vi "HFRR ADV v06.vi"() -> ()   [LabVIEW 2025] (continued)
            n3605 = Concatenate Strings(w4777, w4776, w4778) -> (w4775:string)
            n3606 = Concatenate Strings(w4767, w4768, w4766) -> (w4769:string)
            n3607 = Concatenate Strings(w4764, w4763, w4765) -> (w4762:string)
            n3608 = Concatenate Strings(w4761, w4773, w4790, w4731) -> (w4737:string)
            n3609 = Concatenate Strings(w4761, w4772, w4783, w4731) -> (w4736:string)
            n3610 = Concatenate Strings(w4761, w4771, w4782, w4731) -> (w4735:string)
            n3611 = Concatenate Strings(w4761, w4770, w4775, w4731) -> (w4734:string)
            n3612 = Concatenate Strings(w4761, w4760, w4769, w4731) -> (w4733:string)
            n3613 = Concatenate Strings(w4761, w4759, w4762, "\"}" ("string")) -> (w4732:string)
            n3614 = Concatenate Strings(w4738, w4737, w4736, w4735, w4734, w4733, w4732, "]}" ("string")) -> (w4729:string)
            n3615 = local read "SEN.RUN HRS"() -> (w4696:dbl)
            n3616 = disable-structure shown="Disabled" {
              frame Disabled {
                n3617 = local read "state"() -> (w4815:string[])
                n3618 = Delete From Array(array=w4815, index=0) -> (array with subset deleted=w4813:string[])  [unwired: 1 in, 1 out]
                n3619 = for {
                  N: 6 -> [_]
                  tunnel: w4813 -> [w4826] mode=indexing
                  tunnel: [w4825] -> w4812 mode=indexing
                  n3620 = Equal?(x=w4826, y="Warning") -> (x = y?=w4822:bool)
                  n3621 = Equal?(x=w4826, y="Healthy") -> (x = y?=w4819:bool)
                  n3622 = Select(t="2" ("y"), s=w4822, f="3" ("y")) -> (s? t:f=w4817:string)
                  n3623 = Select(t="1" ("y"), s=w4819, f=w4817) -> (s? t:f=w4825:string)
                }
                "state1" <- w4812
              }
              frame Enabled {
              }
            }
            n3624 = stacked-sequence {
              tunnel: w4729 -> [w4837 _ _]
              tunnel: [_ _ w4853] -> _
              frame #0 {
                (unwired) FALSE ("convert eol (F)")
                w4839 = enum16{"start", "end", "current"}."start" ("pos mode (0:2)")
                n3625 = local read "Path"() -> (w4833:path)
                n3626 = Path To String(path=w4833) -> (string=w4845:string)
                n3627 = Concatenate Strings(w4845, "\\", "Sensor File Name") -> (w4846:string)
                n3628 = local write "standard output 2"(" ") -> ()
                n3629 = String To Path(string=w4846) -> (path=w4836:path)
                n3630 = call <vilib>:"Open_Create_Replace File.vi"("advisory dialog? (display:T)"=FALSE, "function (open:0)"=T23."create or replace", "file path"=w4836) -> ("error out"=w4849:errorcluster, "refnum"=w4848:refnum<file>)  [unwired: 5 in, 2 out]
                n3631 = Set File Position(refnum=w4848, from (0:start)=w4839, error in=w4849) -> (refnum out=w4829:refnum<file>, error out=w4828:errorcluster)  [unwired: 1 in]
                n3632 = Write to Binary File(file (use dialog)=w4829, data=" ", error in=w4828, 5:FALSE ("prepend array or string size? (T)")) -> (refnum out=w4840:refnum<file>, error out=w4841:errorcluster)  [unwired: 2 in, 1 out]
                n3633 = Set File Position(offset (in bytes) (0)=w4839, refnum=w4840, error in=w4841) -> (refnum out=w4832:refnum<file>, error out=w4831:errorcluster)  [unwired: 1 in]
                n3634 = Write to Binary File(file (use dialog)=w4832, data=w4837, error in=w4831, 5:FALSE ("prepend array or string size? (T)")) -> (error out=w4835:errorcluster)  [unwired: 2 in, 2 out]
                n3635 = flat-sequence {
                  tunnel: w4836 -> [w4851]
                  tunnel: w4835 -> [_]
                  frame #0 {
                    n3636 = call <vilib>:"Read Characters From File.vi"("file path (dialog if empty)"=w4851) -> ("character string"=→"Sensor Health JSON string":string)  [unwired: 5 in, 3 out]
                  }
                }
                "SinglePoint  2" <- w4837
              }
              frame #1 {
              }
              frame #2 {
                (unwired) "\"Stored\": true" ("string")
                n3637 = call <vilib>:"System Exec.vi"("run minimized? (F)"=TRUE, "wait until completion? (T)"=TRUE, "working directory"=path "C:/LAB-IQ-NXT", "command line"="C:\\LAB-IQ-NXT\\JPostH.bat") -> ("standard error"=→"Respose From Server 2":string, "standard output"=w4856:string)  [unwired: 4 in, 2 out]
                "standard output 2" <- w4856
                n3638 = Match Pattern(string=w4856, regular expression="JSONH Check String") -> (match substring=w4854:string, offset past match=w4853:i32)  [unwired: 1 in, 2 out]
                n3639 = Equal?(x=w4854, y="JSONH Check String") -> (x = y?=→"Upload \nConfirmed 2":bool)
              }
            }
            n3640 = Divide(x=w4696, y=3600.0 ("f")) -> (x/y=w4689:dbl)
            n3641 = local read "run time"() -> (w4746:string[])
            n3642 = Round To Nearest(number=w4689) -> (nearest integer value=w4688:dbl)
            n3643 = Number To Decimal String(number=w4688) -> (decimal integer string=w4687:string)  [unwired: 1 in]
            n3644 = Index Array(array="Sensor Information", index (col) #1=0 ("disabled index (col)"), index (col) #2=1 ("index (col)"), index (col) #3=2 ("index (col)"), index (col) #4=3 ("index (col)")) -> (element #1=→"Sensor name":string[], element #2=→"model num":string[], element #3=→"run time":string[], element #4=→"state":string[])  [unwired: 4 in]
            n3645 = Insert Into Array(array=w4746, index=1, new element #1=w4687, new element #2=w4687, new element #3=w4687, new element #4=w4687, new element #5=w4687, new element #6=w4687) -> (w4711:string[])
            "run" <- w4711
            n3646 = local read "out"() -> (w4693:string[])
            n3647 = local read "Sensor Information"() -> (w4713:string[][])
            n3648 = Replace Array Subset(array=w4713, new element #1=w4711, index (col) #1=2 ("disabled index (col)"), new element #2=w4693, index (col) #2=3 ("index (col)")) -> (w4712:string[][])  [unwired: 2 in]
            n3649 = local write "Sensor Information"(w4712) -> ()
          }
        }
        n3650 = case shown="True" w4660 {
          frame False {
          }
          frame True {
            n3651 = Equal?(x="FLAG", y=0.0) -> (x = y?=w4677:bool)
            n3652 = case shown="False" w4677 {
              frame False {
                n3653 = Get Date/Time In Seconds() -> (seconds since 1Jan1904=w4683:timestamp)
                n3654 = local read "START 2"() -> (w4681:dbl)
                n3655 = To Double Precision Float(number=w4683) -> (double precision float=w4682:dbl)
                n3656 = Subtract(x=w4682, y=w4681) -> (x-y=→"SENSOR TIME  2":dbl)
              }
              frame True {
                n3657 = Get Date/Time In Seconds() -> (seconds since 1Jan1904=w4685:timestamp)
                n3658 = To Double Precision Float(number=w4685) -> (double precision float=→"START 2":dbl)
                n3659 = local write "FLAG"(100.0 ("FLAG")) -> ()
              }
            }
          }
        }
        n3660 = disable-structure shown="Disabled" {
          disable-tunnel: w4663 -> [w4672 _]
          disable-tunnel: [w4671 _] -> w4662
          frame Disabled {
            n3661 = local read "Json St Flg"() -> (w4670:bool)
            n3662 = case shown="True" w4670 {
              tunnel: w4672 -> [w4673 w4675]
              tunnel: [w4673 w4674] -> w4671
              frame False {
              }
              frame True {
                n3663 = Increment(x=w4675) -> (x+1=w4674:dbl)
                "T cycle" <- w4674
                n3664 = local write "Json St Flg"(FALSE ("Json St Flg")) -> ()
              }
            }
          }
          frame Enabled {
          }
        }
        n3665 = local read "Quit"() -> (w4657:bool)
      }
    }
    frame Enabled {
    }
  }
  n3666 = stacked-sequence {
    tunnel: [w5055] -> w26
    frame #0 {
      w5055 = FALSE ("Upload \nConfirmed")
      n3667 = local write "Upload \nConfirmed"(w5055) -> ()
      n3668 = local write "St Str"("") -> ()
    }
  }
  n3669 = disable-structure shown="Disabled" {
    disable-tunnel: w26 -> [w5056 _]
    frame Disabled {
      n3670 = case shown="True" {
        selector: _ -> [_ _]
        tunnel: w5056 -> [_ w5057]
        frame False {
        }
        frame True {
          n3671 = while {
            tunnel: [w5063] -> _
            tunnel: w5057 -> [_]
            i -> [w5063]
            stop <- w5058 stop-if-true
            n3672 = local read "Json End Flg"() -> (w5062:bool)
            n3673 = Wait (ms)(milliseconds to wait=u32 20 ("Refresh Rate (ms)")) -> ()  [unwired: 1 out]
            n3674 = local read "refresh flag"() -> (w5059:bool)
            n3675 = local read "RUN"() -> (w5060:bool)
            n3676 = And(x=w5060, y=w5059) -> (x .and. y?=w5061:bool)
            n3677 = Or(x=w5061, y=w5062) -> (x .or. y?=w5064:bool)
            "AR Led" <- w5064
            n3678 = case shown="True" w5064 {
              frame False {
              }
              frame True {
                w5081 = "\",\""
                n3679 = local read "UUID"() -> (w5079:string)
                n3680 = local write "refresh flag"(FALSE ("refresh flag")) -> ()
                n3681 = local read "time"() -> (w5068:dbl)
                n3682 = Multiply(x=w5068, y=60.0) -> (x*y=w5067:dbl)
                n3683 = Concatenate Strings("UUID\" : \"", w5079, "\"}") -> (w5082:string)
                n3684 = Number To Fractional String(number=w5067, width (-)=i16 10, precision (6)=i16 4) -> (F-format string=w5096:string)  [unwired: 1 in]
                n3685 = Concatenate Strings("{", "\"Time\":\"", w5096, w5081) -> (w5091:string)
                n3686 = stacked-sequence {
                  tunnel: w5081 -> [w5144 w5152 w5159 w5167 w5175 w5184 w5191]
                  tunnel: [w5145 _ _ _ _ _ _] -> w5095
                  tunnel: [_ w5153 _ _ _ _ _] -> w5094
                  tunnel: [_ _ w5160 _ _ _ _] -> w5093
                  tunnel: [_ _ _ w5169 _ _ _] -> w5092
                  tunnel: w5082 -> [_ _ _ _ _ _ w5202]
                  tunnel: [_ _ _ _ _ _ w5201] -> w5078
                  tunnel: [_ _ _ _ _ w5181 _] -> w5077
                  tunnel: [_ _ _ _ w5174 _ _] -> w5076
                  frame #0 {
                    n3687 = local read "NORMAL LOAD"() -> (w5143:dbl)
                    n3688 = Number To Fractional String(number=w5143, width (-)=i16 10, precision (6)=i16 4) -> (F-format string=w5146:string)  [unwired: 1 in]
                    n3689 = Concatenate Strings("NormalLoad\":\"", w5146, w5144) -> (w5145:string)
                  }
                  frame #1 {
                    n3690 = local read "Temp"() -> (w5151:dbl)
                    n3691 = Number To Fractional String(number=w5151, width (-)=i16 10, precision (6)=i16 4) -> (F-format string=w5154:string)  [unwired: 1 in]
                    n3692 = Concatenate Strings("Temperature\":\"", w5154, w5152) -> (w5153:string)
                  }
                  frame #2 {
                    n3693 = local read "cof"() -> (w5157:dbl)
                    n3694 = Number To Fractional String(number=w5157, width (-)=i16 10, precision (6)=i16 4) -> (F-format string=w5161:string)  [unwired: 1 in]
                    n3695 = Concatenate Strings("FrictionalForce\":\"", w5161, w5159) -> (w5160:string)
                  }
                  frame #3 {
                    n3696 = local read "Set Hz"() -> (w5165:dbl)
                    n3697 = Multiply(x=w5165, y=60.0) -> (x*y=w5164:dbl)
                    n3698 = Number To Fractional String(number=w5164, width (-)=i16 10, precision (6)=i16 4) -> (F-format string=w5170:string)  [unwired: 1 in]
                    n3699 = Concatenate Strings("Speed\":\"", w5170, w5167) -> (w5169:string)
                  }
                  frame #4 {
                    n3700 = local read "Stroke Ln"() -> (w5173:dbl)
                    n3701 = Number To Fractional String(number=w5173, width (-)=i16 10, precision (6)=i16 4) -> (F-format string=w5177:string)  [unwired: 1 in]
                    n3702 = Concatenate Strings("LinearDeformation\":\"", w5177, w5175) -> (w5174:string)
                  }
                  frame #5 {
                    n3703 = local read "AIR TEMP"() -> (w5180:dbl)
                    n3704 = local read "Json St Flg"() -> (w5182:bool)
                    n3705 = local read "Json End Flg"() -> (w5183:bool)
                    n3706 = Number To Fractional String(number=w5180, width (-)=i16 10, precision (6)=i16 4) -> (F-format string=w5186:string)  [unwired: 1 in]
                    n3707 = Concatenate Strings("Vibration\":\"", w5186, w5184) -> (w5181:string)
                    n3708 = And(x=w5182, y=w5183) -> ()  [unwired: 1 out]
                  }
                  frame #6 {
                    n3709 = local read "Json End Flg"() -> (w5190:bool)
                    n3710 = Get Date/Time In Seconds() -> (seconds since 1Jan1904=w5198:timestamp)
                    n3711 = local read "Json St Flg"() -> (w5189:bool)
                    n3712 = To Double Precision Float(number=w5198) -> (double precision float=w5197:dbl)
                    n3713 = Subtract(x=w5197, y=2082844800.0) -> (x-y=w5195:dbl)
                    n3714 = Number To Fractional String(number=w5195, width (-)=i16 12, precision (6)=i16 0) -> (F-format string=w5192:string)  [unwired: 1 in]
                    n3715 = case shown="True" w5190 {
                      tunnel: ["" w5205] -> w5199
                      tunnel: w5192 -> [_ w5206]
                      tunnel: w5191 -> [_ w5204]
                      frame False {
                      }
                      frame True {
                        n3716 = local write "Json End Flg"(FALSE ("Json St Flg")) -> ()
                        n3717 = Concatenate Strings("End\": \"", w5206, w5204) -> (w5205:string)
                      }
                    }
                    n3718 = case shown="True" w5189 {
                      tunnel: [w5209 w5212] -> w5200
                      tunnel: w5192 -> [_ w5213]
                      tunnel: w5191 -> [_ w5210]
                      frame False {
                        n3719 = local read "St Str"() -> (w5209:string)
                      }
                      frame True {
                        n3720 = Concatenate Strings("Start\":\"", w5213, w5210) -> (w5212:string)
                        "St Str" <- w5212
                        n3721 = local write "Json St Flg"(FALSE ("Json St Flg")) -> ()
                      }
                    }
                    n3722 = Concatenate Strings(w5200, w5199, w5202) -> (w5201:string)
                  }
                }
                n3723 = local read "FILE"() -> (w5070:string)
                n3724 = Concatenate Strings("\",\"OperatorID\":\"" ("string"), "Operator ID") -> (w5073:string)
                n3725 = Concatenate Strings("\",\"DatasetTitle\":\"" ("string"), w5070) -> (w5072:string)
                n3726 = Concatenate Strings("\",\"SerialNumber\":\"" ("string"), "Serial No") -> (w5102:string)
                n3727 = Concatenate Strings("\",\"ModelNumber\":\"" ("string"), "Model No") -> (w5101:string)
                n3728 = Concatenate Strings(w5102, w5101) -> (w5084:string)
                n3729 = Concatenate Strings("{\"SecretKey\":\"", "Secret Key", w5084, w5073, w5072, "\",\"Samples\":[") -> (w5089:string)
                n3730 = Concatenate Strings(w5091, w5095, w5094, w5093, w5092, w5076, w5077, w5078) -> (w5090:string)
                n3731 = Concatenate Strings(w5089, w5090, "]}") -> (w5088:string)
                n3732 = stacked-sequence {
                  tunnel: w5088 -> [w5117 _ _]
                  tunnel: [_ _ w5134] -> _
                  frame #0 {
                    (unwired) FALSE ("convert eol (F)")
                    w5119 = enum16{"start", "end", "current"}."start" ("pos mode (0:2)")
                    n3733 = Path To String(path="Path") -> (string=w5125:string)
                    n3734 = Concatenate Strings(w5125, "\\", "Data File Name") -> (w5127:string)
                    n3735 = local write "standard output"(" ") -> ()
                    n3736 = String To Path(string=w5127) -> (path=w5116:path)
                    n3737 = call <vilib>:"Open_Create_Replace File.vi"("advisory dialog? (display:T)"=FALSE, "function (open:0)"=T23."create or replace", "file path"=w5116) -> ("error out"=w5130:errorcluster, "refnum"=w5129:refnum<file>)  [unwired: 5 in, 2 out]
                    n3738 = Set File Position(refnum=w5129, from (0:start)=w5119, error in=w5130) -> (refnum out=w5110:refnum<file>, error out=w5109:errorcluster)  [unwired: 1 in]
                    n3739 = Write to Binary File(file (use dialog)=w5110, data=" ", error in=w5109, 5:FALSE ("prepend array or string size? (T)")) -> (refnum out=w5120:refnum<file>, error out=w5121:errorcluster)  [unwired: 2 in, 1 out]
                    n3740 = Set File Position(offset (in bytes) (0)=w5119, refnum=w5120, error in=w5121) -> (refnum out=w5113:refnum<file>, error out=w5112:errorcluster)  [unwired: 1 in]
                    n3741 = Write to Binary File(file (use dialog)=w5113, data=w5117, error in=w5112, 5:FALSE ("prepend array or string size? (T)")) -> (error out=w5115:errorcluster)  [unwired: 2 in, 2 out]
                    n3742 = flat-sequence {
                      tunnel: w5116 -> [w5132]
                      tunnel: w5115 -> [_]
                      frame #0 {
                        n3743 = call <vilib>:"Read Characters From File.vi"("file path (dialog if empty)"=w5132) -> ("character string"=→"JSON string":string)  [unwired: 5 in, 3 out]
                      }
                    }
                    "SinglePoint" <- w5117
                  }
                  frame #1 {
                  }
                  frame #2 {
                    (unwired) "\"Stored\": true" ("string")
                    n3744 = call <vilib>:"System Exec.vi"("run minimized? (F)"=TRUE, "wait until completion? (T)"=TRUE, "working directory"=path "C:/LAB-IQ-NXT", "command line"="C:\\LAB-IQ-NXT\\JPost.bat") -> ("standard error"=→"Respose From Server":string, "standard output"=w5137:string)  [unwired: 4 in, 2 out]
                    "standard output" <- w5137
                    n3745 = Match Pattern(string=w5137, regular expression="JSON Check String") -> (match substring=w5135:string, offset past match=w5134:i32)  [unwired: 1 in, 2 out]
                    n3746 = Equal?(x=w5135, y="JSON Check String") -> (x = y?=→"Upload \nConfirmed":bool)
                  }
                }
              }
            }
            n3747 = local read "Quit"() -> (w5058:bool)
          }
        }
      }
    }
    frame Enabled {
    }
  }
  n3748 = disable-structure shown="Disabled" {
    disable-tunnel: _ -> [w5220 _]
    frame Disabled {
      n3749 = while {
        shift-right: [w5228] -> w5216
        shift-left: _ -> [w5229]
        shift-right: [w5226] -> w5217
        shift-left: errorcluster {"status"=TRUE, "code"=0, "source"="Init"} ("error out") -> [w5227]
        shift-right: [w5224] -> _
        shift-left: "" -> [w5225]
        tunnel: [w5222] -> _
        tunnel: w5220 -> [_]
        i -> [w5222]
        stop <- w5221 stop-if-true
        n3750 = flat-sequence {
          tunnel: [w5230] -> w5223
          frame #0 {
            n3751 = Wait (ms)(milliseconds to wait=10.0 ("Delay")) -> (millisecond timer value=w5230:u32)
          }
        }
        n3752 = case shown="No Error" w5227 {
          selector: w5227 -> [w5263 w5385]
          tunnel: [w5245 w5387] -> w5228
          tunnel: [w5244 w5386] -> w5226
          tunnel: w5229 -> [w5264 w5379]
          tunnel: w5225 -> [w5243 w5378]
          tunnel: [w5242 w5378] -> w5224
          tunnel: w5223 -> [_ _]
          frame No Error {
            n3753 = Concatenate Strings("COMMAND", "\r", "\n") -> (w5254:string)
            n3754 = case shown="True" "Measure" {
              tunnel: w5264 -> [w5290 w5297]
              tunnel: w5263 -> [w5289 w5296]
              tunnel: [w5290 w5295] -> w5262
              tunnel: [w5289 w5294] -> w5241
              tunnel: w5254 -> [_ w5293]
              frame False {
              }
              frame True {
                n3755 = VISA Write(VISA resource name=w5297, write buffer=w5293, error in (no error)=w5296) -> (VISA resource name out=w5295:refnum<visa-resource-name>, error out=w5294:errorcluster)  [unwired: 1 out]
                n3756 = local write "Read String"("") -> ()
                n3757 = local write "Measure"(FALSE) -> ()
              }
            }
            n3758 = property class="Instr"(reference=w5262, error in=w5241) -> (reference out=w5261:refnum<visa-resource-name>, error out=w5260:errorcluster, "Serial Settings:Number of Bytes at Serial Port"=w5259:u32)
            n3759 = Greater?(x=w5259, y=u32 100) -> (0:w5257:bool)
            n3760 = case shown="True" w5257 {
              tunnel: w5261 -> [w5300 w5325]
              tunnel: w5260 -> [w5299 w5324]
              tunnel: w5259 -> [_ w5323]
              tunnel: [w5300 w5322] -> w5247
              tunnel: [w5299 w5321] -> w5246
              tunnel: w5243 -> [w5298 w5320]
              tunnel: [w5298 ""] -> w5242
              frame False {
              }
              frame True {
                w5310 = u32 6 ("y")
                # "Page 84 of \nmanual"
                n3761 = VISA Read(VISA resource name=w5325, byte count=w5323, error in (no error)=w5324) -> (VISA resource name out=w5322:refnum<visa-resource-name>, read buffer=w5318:string, error out=w5321:errorcluster)  [unwired: 1 out]
                n3762 = while {
                  tunnel: w5318 -> [w5374]
                  tunnel: [w5370] -> w5312 mode=indexing
                  tunnel: [w5364] -> w5316 mode=indexing
                  tunnel: [w5362] -> _
                  i -> [w5362]
                  stop <- w5367 stop-if-true
                  n3763 = String Subset(string=w5374, offset (0)=w5362) -> (substring=w5369:string)  [unwired: 1 in]
                  n3764 = String To Byte Array(string=w5369) -> (unsigned byte array=w5373:u8[])
                  n3765 = String Length(string=w5369) -> (length=w5368:i32)
                  n3766 = Index Array(array=w5373) -> (element=w5372:u8)  [unwired: 1 in]
                  n3767 = Equal To 0?(x=w5368) -> (x = 0?=w5367:bool)
                  n3768 = Number To Boolean Array(number=w5372) -> (Boolean array=w5366:bool[])
                  n3769 = Reverse 1D Array(array=w5366) -> (reversed array=w5365:bool[])
                  n3770 = And(x=w5366, y=bool[] [FALSE, FALSE, FALSE, FALSE, FALSE, FALSE, TRUE, TRUE] ("Boolean array")) -> (x .and. y?=w5370:bool[])
                  n3771 = And(x=w5365, y=bool[] [FALSE, FALSE, TRUE, TRUE, TRUE, TRUE, TRUE, TRUE] ("Boolean array")) -> (x .and. y?=w5364:bool[])
                }
                n3772 = Concatenate Strings(w5320, w5318) -> (→"Read String":string)
                n3773 = while {
                  tunnel: w5312 -> [w5361] mode=indexing
                  tunnel: [w5357] -> w5315
                  i -> [w5357]
                  stop <- w5358 stop-if-true
                  n3774 = Search 1D Array(1D array=w5361, element=TRUE) -> (index of element=w5359:i32)  [unwired: 1 in]
                  n3775 = Less Than 0?(x=w5359) -> (x < 0?=w5358:bool)
                }
                n3776 = Delete From Array(array=w5316, length=w5315, index (row)=0) -> (array with subset deleted=w5311:bool[][])  [unwired: 1 in, 1 out]
                n3777 = Array Size(array=w5311) -> (size(s)=w5313:i32[])
                n3778 = Index Array(array=w5313) -> (element=w5305:i32)  [unwired: 1 in]
                n3779 = Greater?(x=w5305, y=w5310) -> (0:w5308:bool)
                n3780 = Subtract(x=w5305, y=w5310) -> (x-y=w5309:u32)
                n3781 = Select(t=w5309, s=w5308, f=u32 0) -> (s? t:f=w5306:u32)
                n3782 = while {
                  tunnel: w5311 -> [w5344]
                  tunnel: [w5346] -> w5304 mode=indexing
                  tunnel: w5306 -> [w5328]
                  i -> [w5345]
                  stop <- w5343 stop-if-true
                  w5335 = 6 ("index")
                  w5334 = 2 ("length")
                  # "Page 65 of \nmanual"
                  n3783 = Multiply(x=u32 3 ("y"), y=w5345) -> (x*y=w5342:u32)
                  n3784 = Divide(x=u32 102 ("y"), y=u32 65520) -> (x/y=w5352:dbl)
                  n3785 = Greater Or Equal?(x=w5342, y=w5328) -> (x >= y?=w5343:bool)
                  n3786 = Index Array(array=w5344, index (row) #1=w5342) -> (element #1=w5340:bool[], element #2=w5339:bool[], element #3=w5338:bool[])  [unwired: 5 in]
                  n3787 = Reverse 1D Array(array=w5340) -> (reversed array=w5333:bool[])
                  n3788 = Reverse 1D Array(array=w5339) -> (reversed array=w5337:bool[])
                  n3789 = Reverse 1D Array(array=w5338) -> (reversed array=w5336:bool[])
                  n3790 = Delete From Array(array=w5333, length=w5334, index=w5335) -> (array with subset deleted=w5329:bool[])  [unwired: 1 out]
                  n3791 = Delete From Array(array=w5337, length=w5334, index=w5335) -> (array with subset deleted=w5330:bool[])  [unwired: 1 out]
                  n3792 = Delete From Array(array=w5336, length=w5334, index=w5335) -> (array with subset deleted=w5331:bool[])  [unwired: 1 out]
                  n3793 = Insert Into Array(array=bool[] [] ("Boolean array"), new element #1=w5329, new element #2=w5330, new element #3=w5331) -> (w5332:bool[])  [unwired: 1 in]
                  n3794 = Boolean Array To Number(Boolean array=w5332) -> (number=w5341:u32)
                  n3795 = Multiply(x=w5352, y=w5341) -> (x*y=w5351:dbl)
                  n3796 = Decrement(x=w5351) -> (x-1=w5350:dbl)
                  n3797 = Divide(x=w5350, y=u32 100) -> (x/y=w5348:dbl)
                  n3798 = Multiply(x=w5348, y=u32 10) -> (x*y=w5346:dbl)
                }
                n3799 = Delete From Array(array=w5304) -> (array with subset deleted=w5303:dbl[])  [unwired: 2 in, 1 out]
                "Waveform Graph 5" <- w5303
                "Waveform Chart 3" <- w5303
                n3800 = call-poly <vilib>:"Mean.vi"("X"=w5303) -> ("mean"=w5302:dbl)  [unwired: 1 out]
                "Measure_LDS" <- w5302
                n3801 = case shown="True" "Zero 4" {
                  tunnel: w5302 -> [_ w5327]
                  frame False {
                  }
                  frame True {
                    n3802 = local write "Zero 4"(FALSE ("Zero 4")) -> ()
                    "z_measure" <- w5327
                  }
                }
              }
            }
            n3803 = local read "Measure_LDS"() -> (w5237:dbl)
            n3804 = local read "Disp (mm)"() -> (w5236:dbl)
            n3805 = local read "Boolean 7"() -> (w5235:bool)
            n3806 = local read "Boolean 8"() -> (w5234:bool)
            n3807 = case shown="True" "Boolean 8" {
              tunnel: w5236 -> [_ w5267]
              tunnel: w5237 -> [_ w5266]
              frame False {
              }
              frame True {
                n3808 = local read "Captured Values 2"() -> (w5270:dbl[][])
                n3809 = Build Array(w5267, w5266) -> (w5265:dbl[])
                n3810 = Build Array (concatenate)(w5270, w5265) -> (w5268:dbl[][])
                n3811 = local write "Captured Values 2"(w5268) -> ()
                n3812 = local write "Boolean 8"(FALSE ("Boolean 8")) -> ()
              }
            }
            n3813 = call "Build XY Graph"("Enable"=w5234, "Reset"=w5235, "Y Input"=w5237, "X Input"=w5236) -> ("XY Graph"=→"?":cluster{"Y":dbl[], "Y":dbl[]}[])  [unwired: 6 in, 1 out]
            n3814 = case shown="True" "Boolean 9" {
              frame False {
              }
              frame True {
                n3815 = local read "Captured Values 2"() -> (w5272:dbl[][])
                n3816 = Index Array(array=w5272, index (col) #1=0 ("disabled index (col)"), index (col) #2=1 ("index (col)")) -> (element #1=w5275:dbl[], element #2=w5274:dbl[])  [unwired: 2 in]
                n3817 = call <vilib>:"Linear Fit.vi"("Y"=w5275, "X"=w5274) -> ("slope"=→"Slope":dbl, "intercept"=→"Intercept":dbl)  [unwired: 9 in, 3 out]
                n3818 = local write "Boolean 9"(FALSE ("Boolean 9")) -> ()
              }
            }
            n3819 = case shown="True" "Boolean 7" {
              frame False {
              }
              frame True {
                n3820 = local write "Captured Values 2"(dbl[][] [] ("Captured Values")) -> ()
                n3821 = local write "Boolean 7"(FALSE ("Boolean 7")) -> ()
              }
            }
            n3822 = Concatenate Strings("COMMAND 2", "\r", "\n") -> (w5249:string)
            n3823 = case shown="True" "Measure 2" {
              tunnel: w5247 -> [w5282 w5288]
              tunnel: w5246 -> [w5281 w5287]
              tunnel: [w5282 w5286] -> w5245
              tunnel: [w5281 w5285] -> w5244
              tunnel: w5249 -> [_ w5284]
              frame False {
              }
              frame True {
                n3824 = local write "Measure 2"(FALSE ("WRITE")) -> ()
                n3825 = VISA Write(VISA resource name=w5288, write buffer=w5284, error in (no error)=w5287) -> (VISA resource name out=w5286:refnum<visa-resource-name>, error out=w5285:errorcluster)  [unwired: 1 out]
              }
            }
          }
          frame Error {
            w5377 = u16 10 items=["1.0"=10, "1.5"=15, "2.0"=20] ("stop bits (10: 1 bit)")
            n3826 = Wait (ms)(milliseconds to wait=u32 20) -> ()  [unwired: 1 out]
            n3827 = VISA Close(VISA resource name=w5379, error in (no error)=w5385) -> (error out=w5384:errorcluster)
            n3828 = call <vilib>:"Clear Errors.vi"("error in (no error)"=w5384) -> ("error out"=w5383:errorcluster)  [unwired: 5 in, 1 out]
            n3829 = call-poly "VISA Configure Serial Port"("VISA resource name"="Laser Disp Sensor", "timeout (10sec)"=u32 200, "Enable Termination\nChar (T)"=TRUE ("Enable Termination\nChar (T)"), "baud rate (9600)"=u32 921600, "error in (no error)"=w5383, "stop bits (10: 1 bit)"=w5377) -> ("VISA resource name out"=w5387:refnum<visa-resource-name>, "error out"=w5386:errorcluster)  [unwired: 8 in]
          }
        }
        n3830 = local read "Quit"() -> (w5221:bool)
      }
      n3831 = VISA Close(VISA resource name=w5216, error in (no error)=w5217) -> (error out=w5215:errorcluster)
      n3832 = call <vilib>:"Clear Errors.vi"("error in (no error)"=w5215) -> ()  [unwired: 5 in, 2 out]
    }
    frame Enabled {
    }
  }
  n3833 = disable-structure shown="Disabled" {
    disable-tunnel: _ -> [w5392 _]
    frame Disabled {
      n3834 = while {
        tunnel: [w5399] -> _
        shift-right: [w5396] -> w5389
        shift-left: _ -> [w5398]
        shift-right: [w5397] -> w5390
        shift-left: errorcluster {"status"=TRUE, "code"=0, "source"="Init"} ("error out") -> [w5395]
        tunnel: w5392 -> [_]
        i -> [w5399]
        stop <- w5393 stop-if-true
        n3835 = flat-sequence {
          tunnel: w5395 -> [w5490]
          tunnel: [w5490] -> w5394
          frame #0 {
            n3836 = Wait (ms)(milliseconds to wait=u32 50) -> ()  [unwired: 1 out]
          }
        }
        n3837 = case shown="No Error" w5394 {
          selector: w5394 -> [w5440 w5483]
          tunnel: w5398 -> [w5439 w5482]
          tunnel: [w5406 w5473] -> w5397
          tunnel: [w5407 w5481] -> w5396
          frame No Error {
            w5433 = T24 {"Mode"=enum."RTU", "Slave Address"=1} ("Serial Parameters")
            n3838 = call-poly <vilib>:"MB Serial Master Query (poly).vi"("VISA resource name"=w5439, "Starting Address"=i16 1000, "Quantity"=u16 1, "Timeout"=u32 1000, "error in"=w5440, "Serial Parameters"=w5433) -> ("VISA resource name out"=w5434:refnum<visa-resource-name>, "Input Registers"=w5436:u16[], "error out"=w5432:errorcluster)  [unwired: 10 in, 1 out]
            n3839 = Random Number (0-1)() -> (number: 0 to 1=w5421:dbl)
            n3840 = Index Array(array=w5436, index=0) -> (element=w5431:u16)
            n3841 = Subtract(x=w5421, y=0.5) -> (x-y=w5420:dbl)
            n3842 = Divide(x=w5431, y=10 ("index")) -> (x/y=w5425:dbl)
            n3843 = Multiply(x=w5420, y=0.5) -> (x*y=w5419:dbl)
            n3844 = Add(x=w5425, y=w5419) -> (x+y=w5424:dbl)
            n3845 = local read "Amb temp"() -> (w5408:dbl)
            n3846 = Multiply(x=w5424, y=0.2) -> (x*y=w5428:dbl)
            n3847 = Multiply(x=w5408, y=0.8) -> (x*y=w5426:dbl)
            n3848 = Add(x=w5428, y=w5426) -> (x+y=w5409:dbl)
            n3849 = local read "set temp old"() -> (w5403:dbl)
            n3850 = local write "Amb temp"(w5409) -> ()
            n3851 = Select(t="SetTemp 2", s="Heater", f=100.0) -> (s? t:f=w5404:dbl)
            n3852 = Not Equal?(x=w5404, y=w5403) -> (x != y?=w5402:bool)
            n3853 = case shown="True" w5402 {
              tunnel: w5434 -> [w5468 w5470]
              tunnel: [w5467 w5470] -> w5414
              tunnel: w5432 -> [w5466 w5469]
              tunnel: [w5465 w5469] -> w5412
              tunnel: w5404 -> [w5460 _]
              tunnel: w5433 -> [w5462 w5471]
              tunnel: [w5462 w5471] -> w5415
              frame True {
                n3854 = Multiply(x=w5460, y=10 ("index")) -> (x*y=w5459:dbl)
                n3855 = call-poly <vilib>:"MB Serial Master Query (poly).vi"("VISA resource name"=w5468, "Address"=u16 0, "Holding Register"=w5459, "Timeout"=u32 1000, "error in"=w5466, "Serial Parameters"=w5462) -> ("VISA resource name out"=w5467:refnum<visa-resource-name>, "error out"=w5465:errorcluster)  [unwired: 11 in, 1 out]
                "set temp old" <- w5460
              }
              frame False {
              }
            }
            n3856 = flat-sequence {
              tunnel: [w5441] -> _
              tunnel: [w5441] -> w5411
              tunnel: w5412 -> [w5441]
              frame #0 {
                n3857 = Wait (ms)(milliseconds to wait=u32 100) -> ()  [unwired: 1 out]
              }
            }
            n3858 = call "Elapsed Time12"("Time Target (s)"=2.0, "Auto Reset"=TRUE) -> ("Time has Elapsed"=w5416:bool)  [unwired: 10 in, 7 out]
            n3859 = case shown="True" w5416 {
              tunnel: w5415 -> [w5445 w5458]
              tunnel: [w5445 w5458] -> _
              tunnel: [w5444 w5456] -> w5407
              tunnel: w5414 -> [w5444 w5457]
              tunnel: [w5443 w5454] -> w5406
              tunnel: w5411 -> [w5443 w5455]
              frame False {
              }
              frame True {
                n3860 = call-poly <vilib>:"MB Serial Master Query (poly).vi"("VISA resource name"=w5457, "Starting Address"=i16 1003 ("Addr"), "Quantity"=u16 1, "Timeout"=u32 1000, "error in"=w5455, "Serial Parameters"=w5458) -> ("VISA resource name out"=w5456:refnum<visa-resource-name>, "Input Registers"=w5451:u16[], "error out"=w5454:errorcluster)  [unwired: 10 in, 1 out]
                n3861 = Index Array(array=w5451, index=0) -> (element=w5450:u16)
                n3862 = Divide(x=w5450, y=u16 10) -> (x/y=w5446:dbl)
                n3863 = local write "set temp old"(w5446) -> ()
                n3864 = local write "SetTemp"(w5446) -> ()
              }
            }
            "Error Code" <- w5406
            n3865 = Unbundle(w5406) -> ("status"=→"TK4 status":bool)  [unwired: 2 out]
            "SetTemp" <- "SetTemp 2"
          }
          frame Error {
            w5485 = u16 0 items=["None", "Odd", "Even", "Mark", "Space"] ("Parity")
            w5486 = u16 0 items=["None", "XON/XOFF", "RTS/CTS", "XON/XOFF & RTS/CTS", "DTR/DSR", "XON/XOFF & DTR/DSR"] ("Flow Control")
            n3866 = VISA Clear(VISA resource name=w5482, error in (no error)=w5483) -> (VISA resource name out=w5476:refnum<visa-resource-name>, error out=w5474:errorcluster)
            n3867 = VISA Close(VISA resource name=w5476, error in (no error)=w5474) -> (error out=w5475:errorcluster)
            n3868 = call <vilib>:"Clear Errors.vi"("error in (no error)"=w5475) -> ("error out"=w5484:errorcluster)  [unwired: 5 in, 1 out]
            n3869 = Unbundle By Name(T24 {"Mode"=enum."RTU", "Slave Address"=1} ("input cluster")) -> ("Mode"=w5487:enum16{"RTU", "ASCII"})
            n3870 = call <vilib>:"MB Serial Init.vi"("Timeout"=u32 100, "Flow Control"=w5486, "Mode"=w5487, "error in (no error)"=w5484, "Parity"=w5485, "Baud Rate"=u32 9600, "VISA resource name"="Lubrication System COM Port :") -> ("error out"=w5473:errorcluster, "VISA resource name out"=w5481:refnum<visa-resource-name>)  [unwired: 3 in]
            n3871 = local write "set temp old"(0.0 ("set temp old")) -> ()
            n3872 = Unbundle(w5473) -> ("status"=w5472:bool)  [unwired: 2 out]
            n3873 = case shown="True" w5472 {
              selector: w5472 -> [_ w5489]
              frame False {
              }
              frame True {
                n3874 = local write "TK4 status"(w5489) -> ()
              }
            }
          }
        }
        n3875 = local read "Quit"() -> (w5393:bool)
      }
      n3876 = VISA Close(VISA resource name=w5389, error in (no error)=w5390) -> (error out=w5388:errorcluster)
      n3877 = call <vilib>:"Clear Errors.vi"("error in (no error)"=w5388) -> ()  [unwired: 5 in, 2 out]
    }
    frame Enabled {
    }
  }
  "file count" <- 0 ("file count")
